vi "PID_2_Channels_Sequence.vi"() -> ()   [LabVIEW 2016]
uses:
  <vilib>/Analysis/3filter.llb/Filter Passband Type.ctl
  <vilib>/addons/control/pid/pid.llb/PID Advanced (DBL Array).vi
  <vilib>/Analysis/baseanly.llb/Mean (DBL).vi
  <vilib>/addons/control/pid/pid.llb/PID Parameter Manager (DBL Array).vi
  <vilib>/addons/control/pid/pid.llb/PID Derivative Action Buffered (DBL Array).vi
  <vilib>/addons/control/pid/pid.llb/PID Get Advanced Error (DBL Array).vi
  <vilib>/addons/control/pid/pid.llb/PID Integral Action Buffered (DBL Array).vi
  <vilib>/addons/control/pid/pid.llb/PID Resize 1D Array.vi
  <vilib>/addons/control/pid/pid.llb/PID Get Advanced Error (DBL).vi
  <userlib>/Fluigent/Fluigent MFCS/FluigentMFCS_Full.llb/MFCS_EZ Detect.vi
  <userlib>/Fluigent/Fluigent MFCS/FluigentMFCS_Full.llb/MFCS_EZ Initialization.vi
  <userlib>/Fluigent/Fluigent MFCS/FluigentMFCS_Full.llb/MFCS_EZ Write Channel Pressure.vi
  PID2ChanGlobals.vi
  <userlib>/Fluigent/Fluigent MFCS/FluigentMFCS_Full.llb/MFCS_EZ Read Channel Pressure.vi
  <vilib>/Analysis/3filter.llb/Butterworth Filter (DBL).vi
  <vilib>/Analysis/NI_AALBase.lvlib
  <vilib>/addons/control/pid/NI_PID_pid.lvlib
panel:
  in  "Control Pressure Set":dbl=235.0
  in  "Set current pressures to manual pressure":bool
  out "dP/dt":dbl[](graph)
  in  "Fwater (measured)":dbl=600.0
  out "Ratio":dbl[](graph)
  out "F0":dbl[](graph)
  out "Flow Setpoints":dbl[](array[numeric])=[200.784, 133.856]
  in  "Manual Total Mix Flow":dbl=300.0
  out "Total Set Mix Flow":dbl=334.64
  in  "Add Ctrl?":bool=TRUE
  in  "output range":cluster{"output high":dbl, "output low":dbl}[](array[cluster])=[{"output high"=1200.0, "output low"=0.0}] {"output low" format="%.2f"; "output high" format="%.2f"}
  in  "setpoint range":T1(array[cluster])=[{"setpoint high"=1200.0, "setpoint low"=0.0}, {"setpoint high"=1200.0, "setpoint low"=0.0}] {"setpoint high" format="%.2f"; "setpoint low" format="%.2f"}
  in  "Manual Pressure Set":dbl[](array[numeric])=[500.0, 500.0]
  in  "Pressure Channels":enum16{"1", "2", "3", "4"}[](array[ring])=[enum."1", enum."3"]
  in  "gamma":dbl[](array[numeric])=[0.0] format="%.2f"
  in  "linearity":dbl[](array[numeric])=[1.0] format="%.2f"
  in  "beta":dbl[](array[numeric])=[1.0] format="%.2f"
  in  "PID Gains":T2(array[cluster])=[{"Proportional Gain"=0.4, "Integral Time"=0.03, "Derivative Time"=0.0}, {"Proportional Gain"=0.4, "Integral Time"=0.03, "Derivative Time"=0.0}]
  in  "F0 set":dbl=900.0
  out "Current F2":dbl=128.94551724137932
  out "Current F0":dbl=832.3103448275862
  in  "Valves":enum16{"1", "2", "3", "4", "5", "6", "7", "8"}[](array[ring])=[enum."5", enum."4"]
  in  "Boards":enum16{"A", "B", "C"}[](array[ring])=[enum."A", enum."A"]
  out "error out":errorcluster
  out "dt":dbl=0.024001598358154297
  in  "Filter Size":i32=5
  out "Current F1":dbl=200.3448275862069
  in  "reinitialize? (F)":bool
  out "Flow Rates":dbl[][](graph)
  out "Pressure Setpoint":dbl[][](graph)
  in  "stop":bool
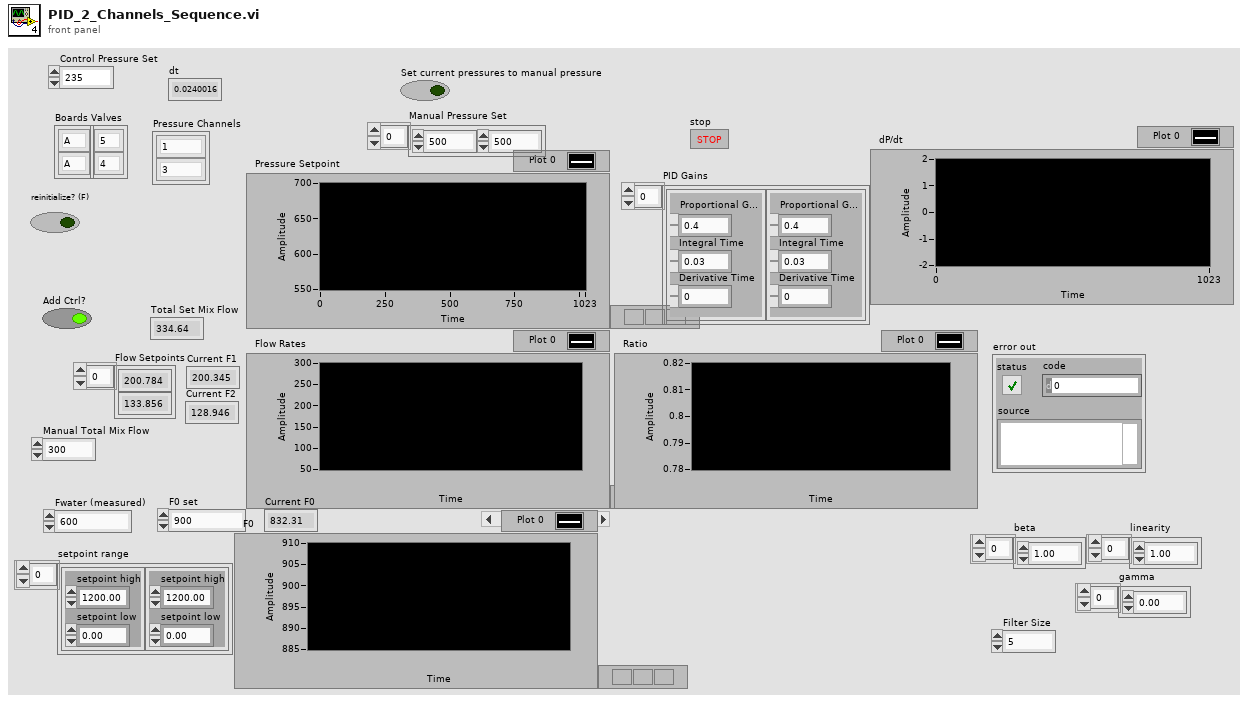
[diagram p1: front panel]
types:
  T1 = cluster{"setpoint high":dbl, "setpoint low":dbl}[]
  T2 = cluster{"Proportional Gain":dbl, "Integral Time":dbl, "Derivative Time":dbl}[]
  T3 = typedef "_EZmfcsSN.ctl" = u16
  T4 = typedef "_EZmfcsRefNum.ctl" = refnum<k1>
  T5 = typedef "_frpRefNum" = refnum<k1>
  T6 = typedef "NI_AALBase.lvlib/Filter Passband Type.ctl" = enum32{"Lowpass", "Highpass", "Bandpass", "Bandstop"}
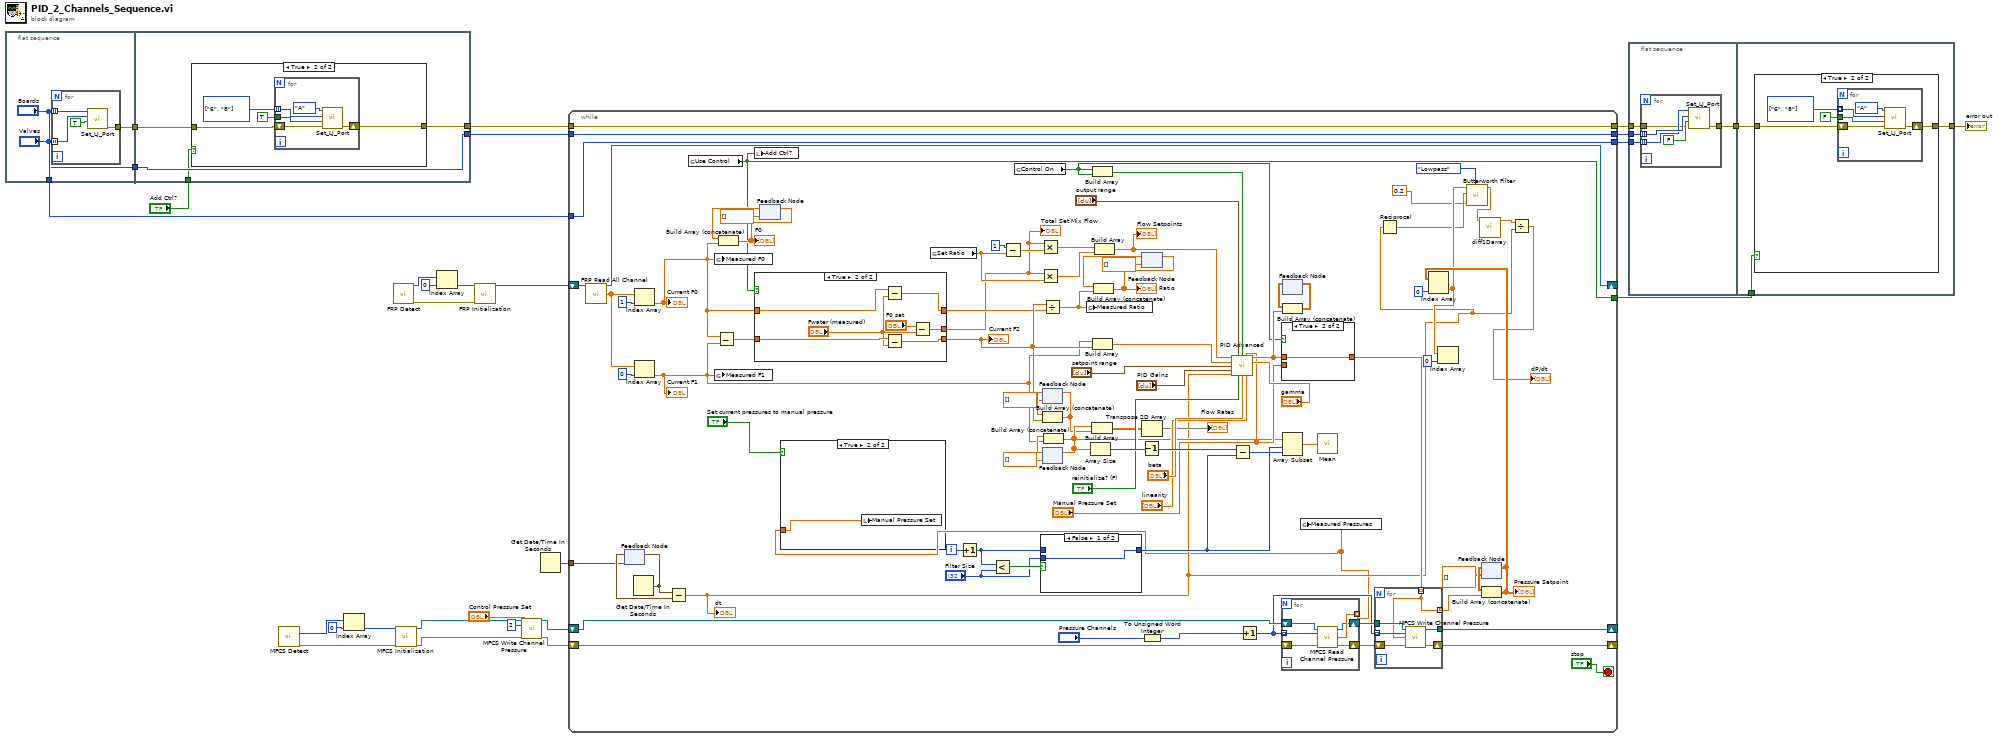
[diagram p0: block diagram]
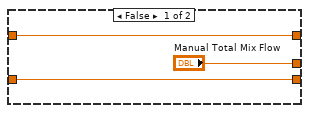
[diagram p5: hidden frame]
diagram:
  n1 = flat-sequence {
    tunnel: ["Boards"] -> w17
    tunnel: [w31] -> w11
    tunnel: ["Valves"] -> w10
    tunnel: [w39] -> w16
    tunnel: [w37] -> w18
    tunnel: w11 -> [w38]
    tunnel: w10 -> [w39]
    tunnel: "Add Ctrl?" -> [w36]
    frame #0 {
      n2 = for {
        tunnel: "Valves" -> [w35] mode=indexing
        tunnel: "Boards" -> [w34] mode=indexing
        tunnel: [w32] -> w31
        n3 = call "Set_LJ_Port.vi"("State"=TRUE, "Channel"=w35, "Flowboard"=w34) -> ("error out"=w32:errorcluster)  [unwired: 8 in]
      }
    }
    frame #1 {
      n4 = case shown="True" w36 {
        tunnel: w38 -> [w40 w44]
        tunnel: [w40 w43] -> w37
        frame False {
        }
        frame True {
          w41 = enum16{"1", "2", "3", "4", "5", "6", "7", "8"}[] [enum."6", enum."8"] items=["1", "2", "3", "4", "5", "6", "7", "8"]
          n5 = for {
            tunnel: TRUE ("State") -> [w47]
            shift-right: [w48] -> w43
            shift-left: w44 -> [w49]
            tunnel: w41 -> [w46] mode=indexing
            n6 = call "Set_LJ_Port.vi"("error in"=w49, "State"=w47, "Channel"=w46, "Flowboard"=enum16{"A", "B", "C"}."A") -> ("error out"=w48:errorcluster)  [unwired: 7 in]
          }
        }
      }
    }
  }
  n7 = call-poly <userlib>:"MFCS Detect.vi"() -> ("[SN MFCS_EZ]"=w28:T3[], "error out"=w26:errorcluster)  [unwired: 14 in]
  n8 = Index Array(array=w28, index=0) -> (element=w27:T3)
  n9 = call <userlib>:"FRP Detect.vi"() -> ("FLOWBOARD List"=w25:u16[], "error out"=w22:errorcluster)  [unwired: 14 in]
  n10 = call-poly <userlib>:"MFCS Initialization.vi"("SN MFCS_EZ"=w27, "error in (no error)"=w26) -> ("MFCS_EZ"=w6:T4, "error out"=w4:errorcluster)  [unwired: 11 in, 1 out]
  n11 = Index Array(array=w25, index=0) -> (element=w21:u16)
  n12 = call <userlib>:"FRP Initialization.vi"("Serial Number"=w21, "error in (no error)"=w22) -> ("FRP out"=w20:T5)  [unwired: 11 in, 2 out]
  n13 = call-poly <userlib>:"MFCS Write Channel Pressure.vi"("MFCS_EZ"=w6, "Channel Number (default=1)"=u8 2, "Pressure (mBar)"="Control Pressure Set", "error in (no error)"=w4) -> ("MFCS_EZ out"=w5:T4, "error out"=w3:errorcluster)  [unwired: 10 in]
  n14 = Get Date/Time In Seconds() -> (seconds since 1Jan1904=w19:timestamp)
  n15 = while {
    shift-right: [w113] -> _
    shift-left: w3 -> [w137]
    shift-right: [w111] -> _
    shift-left: w5 -> [w138]
    shift-right: [w134] -> _
    shift-left: w20 -> [w135]
    tunnel: [w118] -> w13
    tunnel: w18 -> [w118]
    tunnel: w19 -> [w103]
    tunnel: w17 -> [w119]
    tunnel: w16 -> [w120]
    tunnel: [w120] -> w15
    tunnel: [w119] -> w14
    tunnel: [w78] -> w7
    i -> [w129]
    stop <- "stop" stop-if-true
    n16 = call <userlib>:"FRP Read All Channel.vi"("FRP"=w135) -> ("FRP out"=w134:T5, "All Flow-Rates"=w116:dbl[])  [unwired: 12 in, 1 out]
    n17 = feedback #1(w103) -> (w130:timestamp)
    n18 = Get Date/Time In Seconds() -> (seconds since 1Jan1904=w131:timestamp)
    n19 = feedback-in #1(w131) -> ()
    n20 = Index Array(array=w116, index=1) -> (element=w69:dbl)
    "Current F0" <- w69
    n21 = Index Array(array=w116, index=0) -> (element=w68:dbl)
    "Current F1" <- w68
    n22 = Subtract(x=w131, y=w130) -> (x-y=w61:dbl)
    "dt" <- w61
    n23 = global read "PID2ChanGlobals.vi" "Use Control"() -> (w78:bool)
    n24 = global write "PID2ChanGlobals.vi" "Measured F0"(w69) -> ()
    n25 = global write "PID2ChanGlobals.vi" "Measured F1"(w68) -> ()
    n26 = Subtract(x=w69, y=w68) -> (x-y=w91:dbl)
    n27 = local write "Add Ctrl?"(w78) -> ()
    n28 = case shown="True" w78 {
      tunnel: w91 -> [w142 w149]
      tunnel: [w142 w148] -> w83
      tunnel: ["Manual Total Mix Flow" w144] -> w70
      tunnel: w69 -> [w140 w147]
      tunnel: [w140 w146] -> w82
      frame False {
      }
      frame True {
        n29 = Subtract(x=w147, y="Fwater (measured)") -> (x-y=w146:dbl)
        n30 = Subtract(x=w149, y="Fwater (measured)") -> (x-y=w148:dbl)
        n31 = Subtract(x="F0 set", y="Fwater (measured)") -> (x-y=w144:dbl)
      }
    }
    "Current F2" <- w83
    "Total Set Mix Flow" <- w70
    n32 = feedback #2(dbl[] []) -> (w84:dbl[])
    n33 = Build Array (concatenate)(w84, w69) -> (w85:dbl[])
    "F0" <- w85
    n34 = feedback-in #2(w85) -> ()
    n35 = global read "PID2ChanGlobals.vi" "Set Ratio"() -> (w71:dbl)
    n36 = Increment(x=w129) -> (x+1=w127:i32)
    n37 = Less?(x=w127, y="Filter Size") -> (x < y?=w128:bool)
    n38 = Subtract(x=1, y=w71) -> (x-y=w89:dbl)
    n39 = global read "PID2ChanGlobals.vi" "Control On"() -> (w76:bool)
    n40 = Multiply(x=w70, y=w89) -> (x*y=w88:dbl)
    n41 = Multiply(x=w70, y=w71) -> (x*y=w87:dbl)
    n42 = case shown="False" w128 {
      tunnel: w127 -> [_ w165]
      tunnel: [w164 w165] -> w124
      tunnel: "Filter Size" -> [w164 _]
      frame False {
      }
      frame True {
      }
    }
    n43 = Divide(x=w83, y=w82) -> (x/y=w81:dbl)
    n44 = feedback #3(dbl[] []) -> (w102:dbl[])
    n45 = Build Array (concatenate)(w102, w83) -> (w74:dbl[])
    n46 = feedback-in #3(w74) -> ()
    n47 = feedback #4(dbl[] []) -> (w132:dbl[])
    n48 = Build Array (concatenate)(w132, w68) -> (w75:dbl[])
    n49 = feedback-in #4(w75) -> ()
    n50 = global write "PID2ChanGlobals.vi" "Measured Ratio"(w81) -> ()
    n51 = Array Size(array=w75) -> (size(s)=w125:i32)
    n52 = Build Array(w75, w74) -> (w73:dbl[][])
    n53 = Build Array(w76, w76) -> (w77:bool[])
    n54 = Build Array(w68, w83) -> (w93:dbl[])
    n55 = Build Array(w88, w87) -> (w86:dbl[])
    "Flow Setpoints" <- w86
    n56 = feedback #5(dbl[] []) -> (w80:dbl[])
    n57 = Build Array (concatenate)(w80, w81) -> (w79:dbl[])
    "Ratio" <- w79
    n58 = feedback-in #5(w79) -> ()
    n59 = Transpose 2D Array(2D array=w73) -> (transposed array=→"Flow Rates":dbl[][])
    n60 = Decrement(x=w125) -> (x-1=w123:i32)
    n61 = To Unsigned Word Integer(number="Pressure Channels") -> (unsigned 16bit integer=w101:u16[])
    n62 = call-poly <vilib>:"PID Advanced.vi"("setpoint"=w86, "output range"="output range", "auto? (T)"=w77, "manual control"="Manual Pressure Set", "process variable"=w93, "gamma"="gamma", "setpoint range"="setpoint range", "PID gains"="PID Gains", "dt (s)"=w61, "reinitialize? (F)"="reinitialize? (F)", "beta"="beta", "linearity"="linearity") -> ("output"=w96:dbl[])  [unwired: 2 in, 1 out]
    n63 = Subtract(x=w123, y=w124) -> (x-y=w122:i32)
    n64 = Increment(x=w101) -> (x+1=w104:u16[])
    n65 = case shown="True" w76 {
      tunnel: "Manual Pressure Set" -> [w150 _]
      tunnel: [w150 w151] -> w97
      tunnel: w96 -> [_ w151]
      frame False {
      }
      frame True {
      }
    }
    n66 = for {
      tunnel: [w155] -> w50 mode=indexing
      shift-right: [w154] -> w115
      shift-left: w138 -> [w157]
      shift-right: [w153] -> w114
      shift-left: w137 -> [w156]
      tunnel: w104 -> [w152] mode=indexing
      n67 = call-poly <userlib>:"MFCS Read Channel Pressure.vi"("MFCS_EZ"=w157, "Channel Number (default=1)"=w152, "error in (no error)"=w156) -> ("MFCS_EZ out"=w154:T4, "Pressure (mBar)"=w155:dbl, "error out"=w153:errorcluster)  [unwired: 9 in, 1 out]
    }
    n68 = case shown="True" "Set current pressures to manual pressure" {
      tunnel: w50 -> [_ w139]
      frame False {
      }
      frame True {
        n69 = local write "Manual Pressure Set"(w139) -> ()
      }
    }
    n70 = feedback #6() -> (w100:dbl[][])  [unwired: 1 in]
    n71 = Build Array (concatenate)(w100, w96) -> (w99:dbl[][])
    n72 = feedback-in #6(w99) -> ()
    n73 = Array Subset(array=w75, index=w122, length=w124) -> (w121:dbl[])
    n74 = global write "PID2ChanGlobals.vi" "Measured Pressures"(w50) -> ()
    n75 = call-poly <vilib>:"Mean.vi"("X"=w121) -> ()  [unwired: 2 out]
    n76 = for {
      tunnel: w115 -> [w163]
      shift-right: [w161] -> w113
      shift-left: w114 -> [w162]
      tunnel: [w158] -> w94 mode=indexing
      tunnel: [w160] -> w111
      tunnel: w104 -> [w159] mode=indexing
      tunnel: w97 -> [w158] mode=indexing
      n77 = call-poly <userlib>:"MFCS Write Channel Pressure.vi"("MFCS_EZ"=w163, "Channel Number (default=1)"=w159, "Pressure (mBar)"=w158, "error in (no error)"=w162) -> ("MFCS_EZ out"=w160:T4, "error out"=w161:errorcluster)  [unwired: 10 in]
    }
    n78 = Reciprocal(x=w61) -> (1/x=w60:dbl)
    n79 = feedback #7(dbl[][] []) -> (w112:dbl[][])
    n80 = Build Array (concatenate)(w112, w94) -> (w67:dbl[][])
    "Pressure Setpoint" <- w67
    n81 = Index Array(array=w67, index (col)=0 ("disabled index (col)")) -> (element=w62:dbl[])  [unwired: 1 in]
    n82 = Index Array(array=w62, index=0) -> ()  [unwired: 1 out]
    n83 = call-poly <vilib>:"Butterworth Filter.vi"("filter type"=Filter_Passband_Type."Lowpass", "low cutoff freq: fl"=0.2 ("high cutoff freq: fh"), "sampling freq: fs"=w60, "X"=w62) -> ("Filtered X"=w57:dbl[])  [unwired: 4 in, 1 out]
    n84 = call "diff1Darray.vi"("Input"=w57) -> ("Diff"=w64:dbl[])  [unwired: 10 in]
    n85 = feedback-in #7(w67) -> ()
    n86 = Divide(x=w64, y=w61) -> (x/y=→"dP/dt":dbl[])
  }
  n87 = flat-sequence {
    tunnel: w15 -> [w169]
    tunnel: w14 -> [w168]
    tunnel: w13 -> [w167]
    tunnel: [w166] -> w8
    tunnel: [w176] -> w12
    tunnel: w8 -> [w175]
    tunnel: w7 -> [w177]
    frame #0 {
      n88 = for {
        tunnel: w169 -> [w174] mode=indexing
        tunnel: [w172] -> w166
        tunnel: w168 -> [w171] mode=indexing
        tunnel: w167 -> [w170]
        n89 = call "Set_LJ_Port.vi"("error in"=w170, "State"=FALSE, "Channel"=w174, "Flowboard"=w171) -> ("error out"=w172:errorcluster)  [unwired: 7 in]
      }
    }
    frame #1 {
      n90 = case shown="True" w177 {
        tunnel: w175 -> [w178 w179]
        tunnel: [w178 w182] -> w176
        frame False {
        }
        frame True {
          w180 = enum16{"1", "2", "3", "4", "5", "6", "7", "8"}[] [enum."6", enum."8"] items=["1", "2", "3", "4", "5", "6", "7", "8"]
          n91 = for {
            tunnel: FALSE ("State") -> [w185]
            shift-right: [w186] -> w182
            shift-left: w179 -> [w187]
            tunnel: w180 -> [w184] mode=indexing
            n92 = call "Set_LJ_Port.vi"("error in"=w187, "State"=w185, "Channel"=w184, "Flowboard"=enum16{"A", "B", "C"}."A") -> ("error out"=w186:errorcluster)  [unwired: 7 in]
          }
        }
      }
    }
  }
  "error out" <- w12
